vi "_emi_GFV Debug Log.vi"(1 "Action(GET)":enum16{"GET", "SET"}(ring), 7 "Debug Log":bool, 11 "error in (no error)":errorcluster) -> (8 "Debug Log out":bool, 15 "error out":errorcluster)   [LabVIEW 2011]
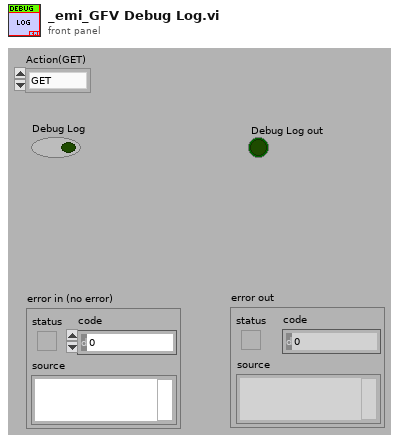
[diagram p1: front panel]
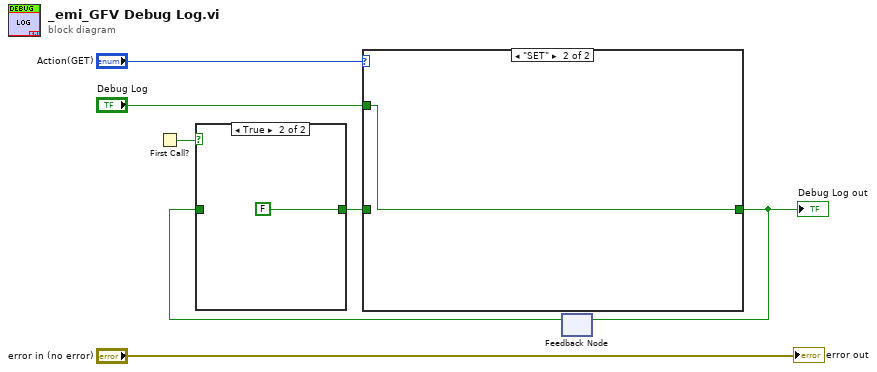
[diagram p0: block diagram]
diagram:
  n1 = First Call?() -> (First Call?: T/F=w4:bool)
  n2 = feedback #1() -> (w5:bool)  [unwired: 1 in]
  n3 = case shown="True" w4 {
    tunnel: w5 -> [w8 _]
    tunnel: [w8 FALSE] -> w2
    frame False {
    }
    frame True {
    }
  }
  n4 = case shown="\"SET\"" "Action(GET)" {
    tunnel: [w10 w11] -> w3
    tunnel: w2 -> [w10 _]
    tunnel: "Debug Log" -> [_ w11]
    frame "GET", Default {
    }
    frame "SET" {
    }
  }
  "Debug Log out" <- w3
  n5 = feedback-in #1(w3) -> ()
  "error out" <- "error in (no error)"
